vi "SetPersistentConfiguration.vi"(8 "ErrorIn":errorcluster, 9 "DataIn":variant, 11 "ReferenceIn":refnum<class "TemplateGUI.lvclass">) -> (0 "ErrorOut":errorcluster, 1 "DataOut":variant, 3 "ReferenceOut":refnum<class "TemplateGUI.lvclass">)   [LabVIEW 2021, in "TemplateGUIOpenGDSActiveObject.lvlib" / "TemplateGUI.lvclass"]
doc: "Sets the persistent data in the object"
uses:
  TemplateGUI.lvclass
  a2d9dd7e-4f73-47a2-b010-087cab1955c7.vi
  <vilib>/Utility/LVClass/Get LV Class Name.vi
  Library_TAF_ApplicationFramework/TAFBaseGUI/TAFBaseGUI.lvclass
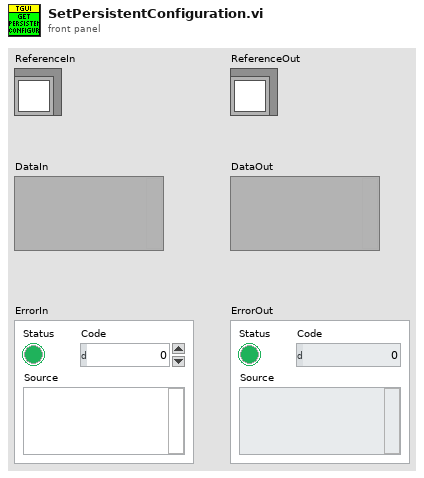
[diagram p1: front panel]
types:
  T1 = typedef "TemplateGUI.lvlib/TemplateGUI.lvclass/ObjectAttributes.ctl" = cluster{"Interfaces":cluster{"Dummys":refnum<class>}, "Locals":cluster{"MainGUIActive":refnum<queue>}, "Persistent":cluster{"Dummy":bool}}
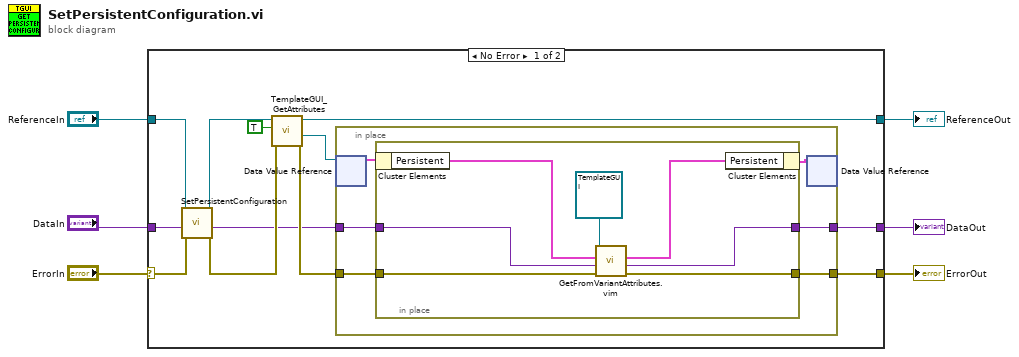
[diagram p0: block diagram]
diagram:
  n1 = case shown="No Error" "ErrorIn" {
    selector: "ErrorIn" -> [w16 w34]
    tunnel: [w17 w34] -> w5
    tunnel: [w14 w33] -> w3
    tunnel: "ReferenceIn" -> [w7 w33]
    tunnel: [w13 w32] -> w2
    tunnel: "DataIn" -> [w9 w32]
    frame No Error {
      n2 = call-parent "SetPersistentConfiguration.vi"("ErrorIn"=w16, "DataIn"=w9, "ReferenceIn"=w7) -> ("ErrorOut"=w15:errorcluster, "DataOut"=w10:variant, "ReferenceOut"=w8:refnum<class "TemplateGUI.lvclass">)  [unwired: 6 in]
      n3 = call "TemplateGUI_GetAttributes.vi"("ErrorIn"=w15, "OnlyGetDvrReference(False)"=TRUE, "ReferenceIn"=w8) -> ("ErrorOut"=w18:errorcluster, "DataRef"=w11:refnum<data-value>, "ReferenceOut"=w14:refnum<class "TemplateGUI.lvclass">)  [unwired: 5 in, 1 out]
      n4 = in-place {
        in-place-border: w18 -> [w24]
        in-place-border: [w23] -> w17
        in-place-border: w10 -> [w22]
        in-place-border: [w21] -> w13
        n5 = in-place-dvr #1(w11) -> (w20:T1)  [unwired: 1 out]
        n6 = in-place {
          in-place-border: w24 -> [w31]
          in-place-border: [w30] -> w23
          in-place-border: w22 -> [w29]
          in-place-border: [w28] -> w21
          n7 = in-place-cluster #2(w20) -> ("Persistent"=w26:cluster{"Dummy":bool})
          n8 = call "GetFromVariantAttributes.vim"("ErrorIn"=w31, "DataInIn"=w29, "PersistentDataType"=w26, "Object"=refnum<class "TemplateGUI.lvclass"> refnum ("VerticalButtonBar")) -> ("ErrorOut"=w30:errorcluster, "DataOut"=w28:variant, "PersistentDataOut"=w25:cluster{"Dummy":bool})  [unwired: 5 in]
          n9 = in-place-cluster #2("Persistent"=w25) -> (w19:T1)
        }
        n10 = in-place-dvr #1(w19) -> ()  [unwired: 2 out]
      }
    }
    frame Error {
    }
  }
  "ErrorOut" <- w5
  "ReferenceOut" <- w3
  "DataOut" <- w2
